vi "ScanSensor_01_10_19.vi"() -> ()   [LabVIEW 2016]
uses:
  <instrlib>/Keyence LK-G3000/Public/enums/LKIF_OUTNO.ctl
  <vilib>/Utility/file.llb/Write Delimited Spreadsheet (DBL).vi
  <instrlib>/Keyence LK-G3000/Keyence LK-G3000.lvlib
panel:
  out "z-axis":dbl
  out "x = y?":bool
  in  "Speed":dbl=5.0
  in  "Distance":dbl=0.05
  out "Position Feedback":dbl
  in  "AxisName":string="Z"
  out "R^2 Bottom Sensor":dbl
  out "RMSE Bottom Sensor":dbl
  out "R^2 Top Sensor":dbl
  out "RMSE Top Sensor":dbl
  out "Microradians":dbl format="%#_7g"
  out "Z Position":string
  out "Y Position":string
  out "X Axis Position":string
  out "Z Home Position":string
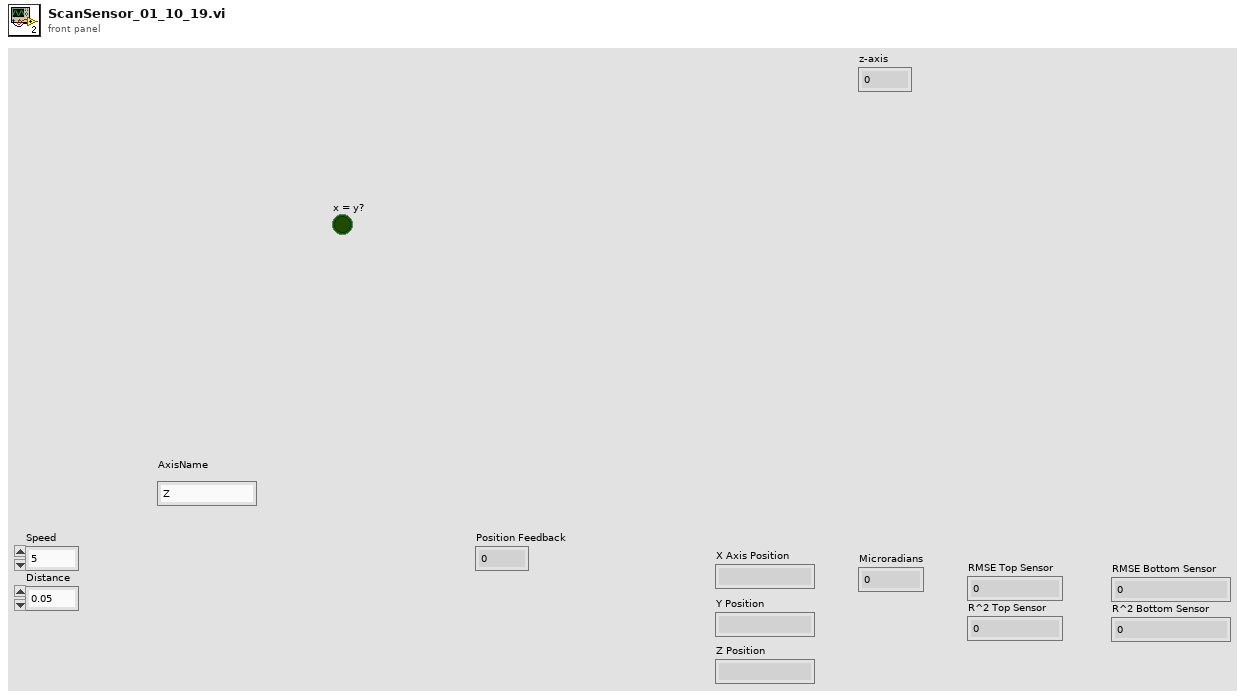
[diagram p1: front panel]
types:
  T1 = typedef "Keyence LK-G3000.lvlib/LKIF_FLOATVALUE.ctl" = cluster{"LKIF_FLOATRESULT":T2, "Value":sgl}
  T2 = typedef "Keyence LK-G3000.lvlib/LKIF_FLOATRESULT.ctl" = i32
  T3 = typedef "Keyence LK-G3000.lvlib/LKIF_OUTNO.ctl" = i32
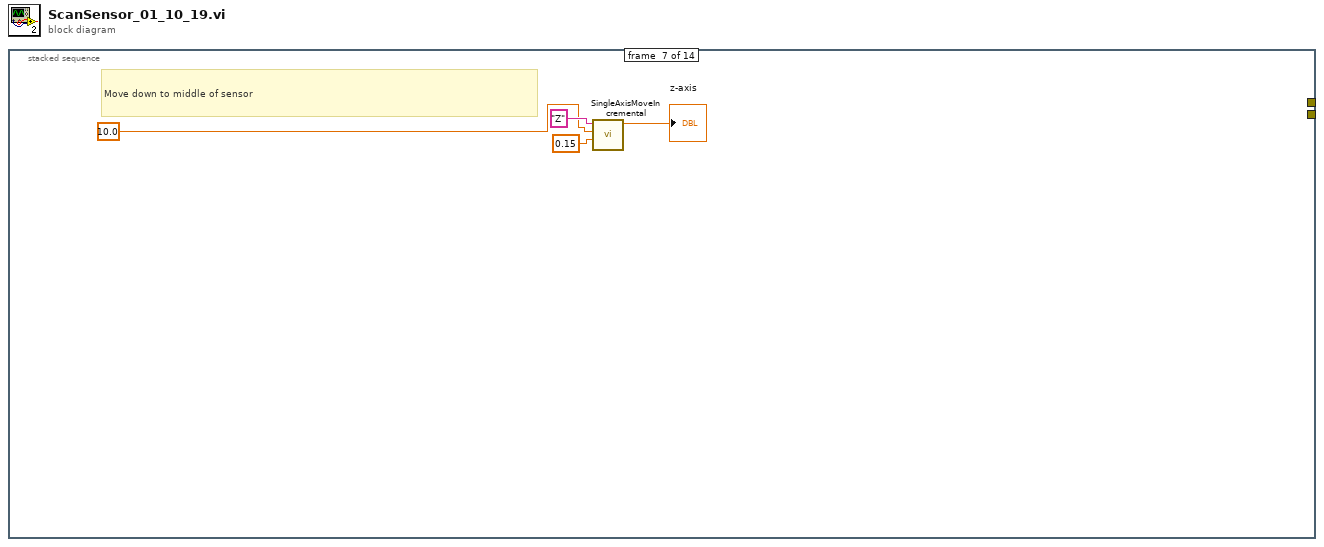
[diagram p0: block diagram]
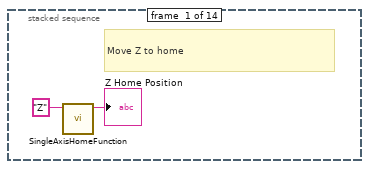
[diagram p2: hidden frame]
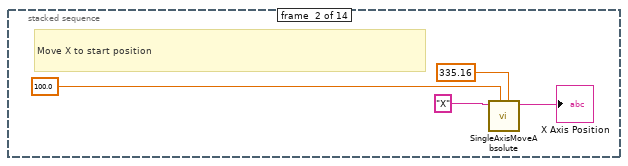
[diagram p3: hidden frame]
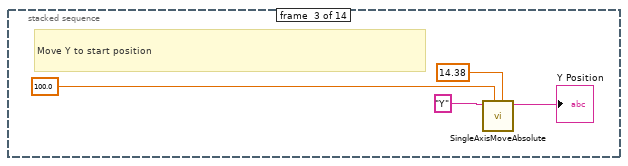
[diagram p4: hidden frame]
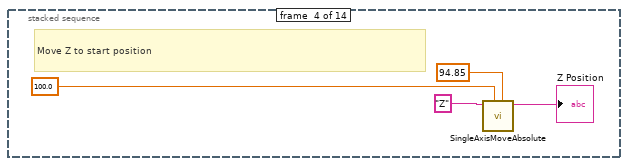
[diagram p5: hidden frame]
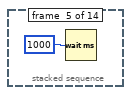
[diagram p6: hidden frame]
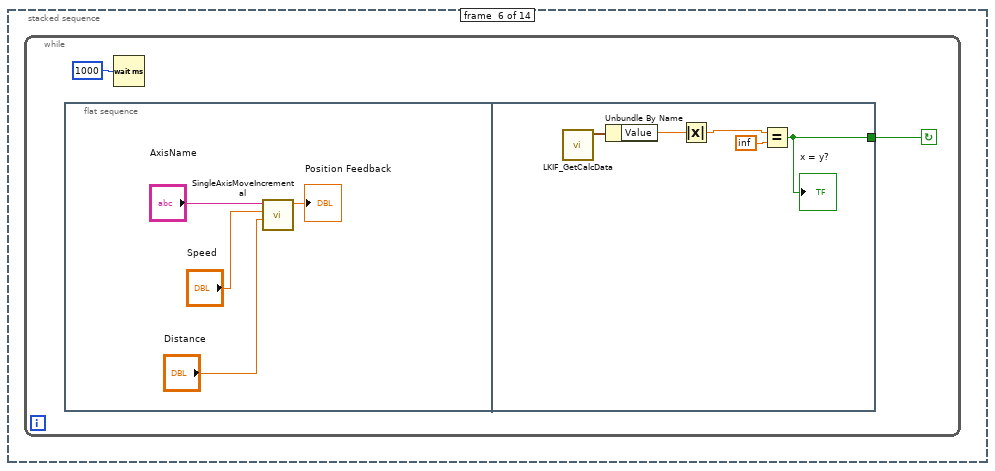
[diagram p7: hidden frame]
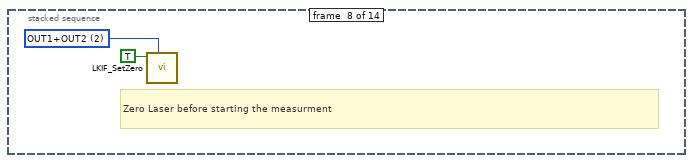
[diagram p8: hidden frame]
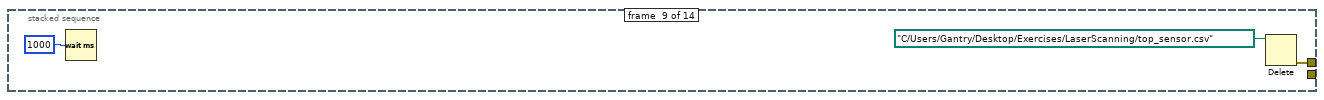
[diagram p9: hidden frame]
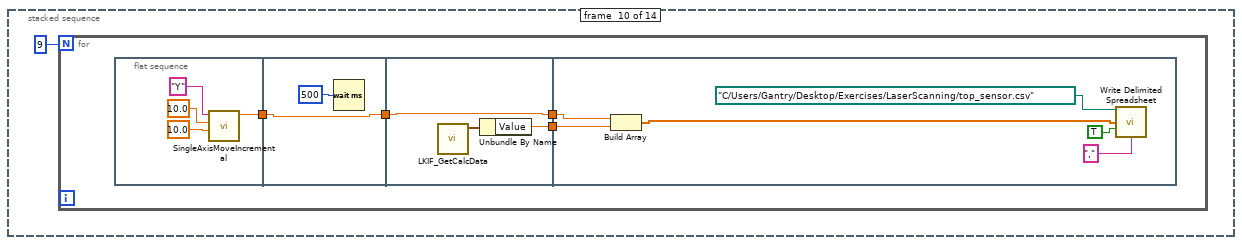
[diagram p10: hidden frame]
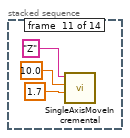
[diagram p11: hidden frame]
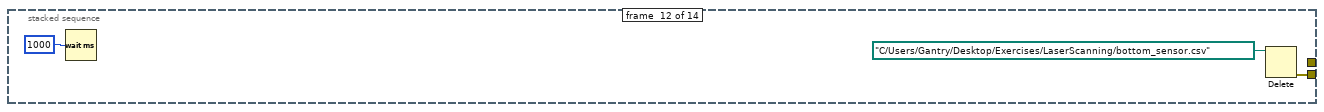
[diagram p12: hidden frame]
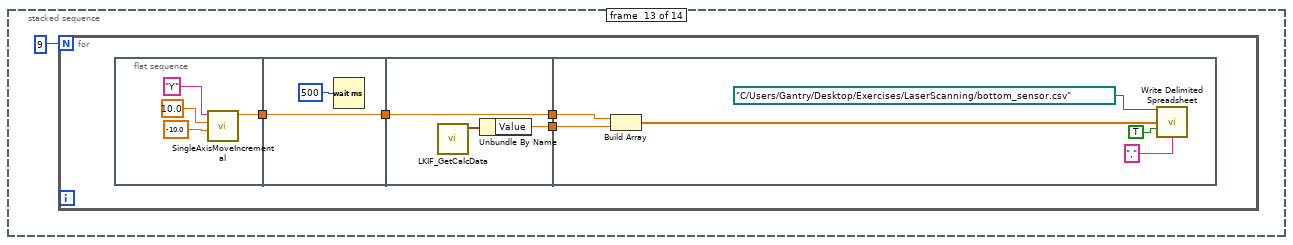
[diagram p13: hidden frame]
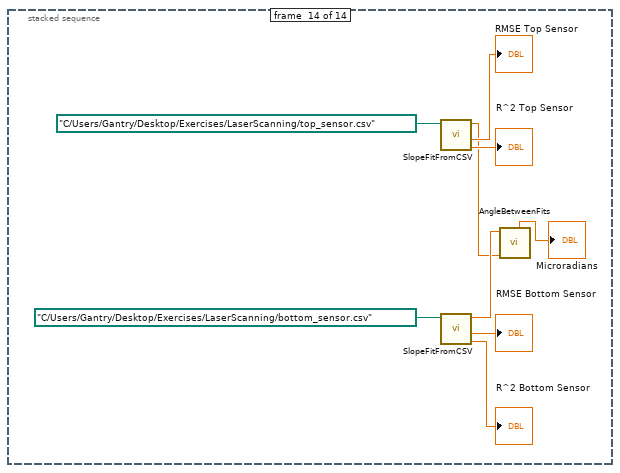
[diagram p14: hidden frame]
diagram:
  n1 = stacked-sequence {
    tunnel: [_ _ _ _ _ _ _ _ w33 _ _ _ _ _] -> _
    tunnel: [_ _ _ _ _ _ _ _ _ _ _ w59 _ _] -> _
    frame #0 {
      # "Move Z to home"
      n2 = call "SingleAxisHomeFunction.vi"("AxisName"="Z") -> ("Position"=→"Z Home Position":string)  [unwired: 10 in]
    }
    frame #1 {
      # "Move X to start position"
      n3 = call "SingleAxisMoveAbsolute.vi"("Position"=335.16, "Speed"=100.0, "AxisName"="X") -> ("Axis Position"=→"X Axis Position":string)  [unwired: 8 in]
    }
    frame #2 {
      # "Move Y to start position"
      n4 = call "SingleAxisMoveAbsolute.vi"("Position"=14.38, "Speed"=100.0, "AxisName"="Y") -> ("Axis Position"=→"Y Position":string)  [unwired: 8 in]
    }
    frame #3 {
      # "Move Z to start position"
      n5 = call "SingleAxisMoveAbsolute.vi"("Position"=94.85, "Speed"=100.0, "AxisName"="Z") -> ("Axis Position"=→"Z Position":string)  [unwired: 8 in]
    }
    frame #4 {
      n6 = Wait (ms)(milliseconds to wait=u32 1000) -> ()  [unwired: 1 out]
    }
    frame #5 {
      n7 = while {
        stop <- w16 continue-if-true
        n8 = flat-sequence {
          tunnel: [w22] -> w16
          frame #0 {
            n9 = call "SingleAxisMoveIncremental.vi"("Distance"="Distance", "Speed"="Speed", "AxisName"="AxisName") -> ("Position Feedback"=→"Position Feedback":dbl)  [unwired: 8 in]
          }
          frame #1 {
            n10 = call <instrlib>:"LKIF_GetCalcData.vi"() -> ("CalcData1"=w23:T1)  [unwired: 9 in, 2 out]
            n11 = Unbundle By Name(w23) -> ("Value"=w24:sgl)
            n12 = Absolute Value(x=w24) -> (abs(x)=w25:sgl)
            n13 = Equal?(x=w25, y=inf) -> (x = y?=w22:bool)
            "x = y?" <- w22
          }
        }
        n14 = Wait (ms)(milliseconds to wait=u32 1000) -> ()  [unwired: 1 out]
      }
    }
    frame #6 {
      # "Move down to middle of sensor"
      n15 = call "SingleAxisMoveIncremental.vi"("Distance"=0.15 ("Position"), "Speed"=10.0, "AxisName"="Z") -> ("Position Feedback"=→"z-axis":dbl)  [unwired: 8 in]
    }
    frame #7 {
      w32 = T3 2 items=["OUT1", "OUT2", "OUT1+OUT2"] ("OutNo (OUT1)")
      # "Zero Laser before starting the measurment"
      n16 = call <instrlib>:"LKIF_SetZero.vi"("OutNo (OUT1)"=w32, "IsOn"=TRUE) -> ()  [unwired: 9 in, 1 out]
    }
    frame #8 {
      n17 = Wait (ms)(milliseconds to wait=u32 1000) -> ()  [unwired: 1 out]
      n18 = Delete(path (use dialog)=path "C:/Users/Gantry/Desktop/Exercises/LaserScanning/top_sensor.csv") -> (error out=w33:errorcluster)  [unwired: 4 in, 2 out]
    }
    frame #9 {
      n19 = for {
        N: 9 -> [_]
        n20 = flat-sequence {
          tunnel: [w41] -> w38
          tunnel: [w45] -> w39
          tunnel: w38 -> [w45]
          tunnel: [w48] -> w40
          tunnel: w39 -> [w48]
          tunnel: [w47] -> w37
          tunnel: w40 -> [w55]
          tunnel: w37 -> [w54]
          frame #0 {
            n21 = call "SingleAxisMoveIncremental.vi"("Distance"=10.0, "Speed"=10.0, "AxisName"="Y") -> ("Position Feedback"=w41:dbl)  [unwired: 8 in]
          }
          frame #1 {
            n22 = Wait (ms)(milliseconds to wait=u32 500) -> ()  [unwired: 1 out]
          }
          frame #2 {
            n23 = call <instrlib>:"LKIF_GetCalcData.vi"() -> ("CalcData1"=w49:T1)  [unwired: 9 in, 2 out]
            n24 = Unbundle By Name(w49) -> ("Value"=w47:sgl)
          }
          frame #3 {
            n25 = Build Array(w55, w54) -> (w53:dbl[])
            n26 = call-poly <vilib>:"Write Delimited Spreadsheet.vi"("file path (dialog if empty)"=path "C:/Users/Gantry/Desktop/Exercises/LaserScanning/top_sensor.csv", "1D data"=w53, "append to file? (new file:F)"=TRUE, "delimiter (\\t)"="," ("delimiter (\\t)")) -> ()  [unwired: 10 in, 2 out]
          }
        }
      }
    }
    frame #10 {
      n27 = call "SingleAxisMoveIncremental.vi"("Distance"=1.7, "Speed"=10.0, "AxisName"="Z") -> ()  [unwired: 8 in, 1 out]
    }
    frame #11 {
      n28 = Wait (ms)(milliseconds to wait=u32 1000) -> ()  [unwired: 1 out]
      n29 = Delete(path (use dialog)=path "C:/Users/Gantry/Desktop/Exercises/LaserScanning/bottom_sensor.csv") -> (error out=w59:errorcluster)  [unwired: 4 in, 2 out]
    }
    frame #12 {
      n30 = for {
        N: 9 -> [_]
        n31 = flat-sequence {
          tunnel: [w67] -> w64
          tunnel: [w71] -> w65
          tunnel: w64 -> [w71]
          tunnel: [w74] -> w66
          tunnel: w65 -> [w74]
          tunnel: [w73] -> w63
          tunnel: w66 -> [w81]
          tunnel: w63 -> [w80]
          frame #0 {
            n32 = call "SingleAxisMoveIncremental.vi"("Distance"=-10.0, "Speed"=10.0, "AxisName"="Y") -> ("Position Feedback"=w67:dbl)  [unwired: 8 in]
          }
          frame #1 {
            n33 = Wait (ms)(milliseconds to wait=u32 500) -> ()  [unwired: 1 out]
          }
          frame #2 {
            n34 = call <instrlib>:"LKIF_GetCalcData.vi"() -> ("CalcData1"=w75:T1)  [unwired: 9 in, 2 out]
            n35 = Unbundle By Name(w75) -> ("Value"=w73:sgl)
          }
          frame #3 {
            n36 = Build Array(w81, w80) -> (w79:dbl[])
            n37 = call-poly <vilib>:"Write Delimited Spreadsheet.vi"("file path (dialog if empty)"=path "C:/Users/Gantry/Desktop/Exercises/LaserScanning/bottom_sensor.csv", "1D data"=w79, "append to file? (new file:F)"=TRUE, "delimiter (\\t)"="," ("delimiter (\\t)")) -> ()  [unwired: 10 in, 2 out]
          }
        }
      }
    }
    frame #13 {
      n38 = call "SlopeFitFromCSV.vi"("file path"=path "C:/Users/Gantry/Desktop/Exercises/LaserScanning/top_sensor.csv") -> ("R-square"=→"R^2 Top Sensor":dbl, "RMSE"=→"RMSE Top Sensor":dbl, "slope"=w82:dbl)  [unwired: 7 in, 1 out]
      n39 = call "SlopeFitFromCSV.vi"("file path"=path "C:/Users/Gantry/Desktop/Exercises/LaserScanning/bottom_sensor.csv") -> ("R-square"=→"R^2 Bottom Sensor":dbl, "RMSE"=→"RMSE Bottom Sensor":dbl, "slope"=w83:dbl)  [unwired: 7 in, 1 out]
      n40 = call "AngleBetweenFits.vi"("Slope 2"=w82, "Slope 1"=w83) -> ("Microradians"=→"Microradians":dbl)  [unwired: 9 in]
    }
  }
